vi "Actor Receive.vi"(11 "Dev Actor in":refnum<class "Dev Actor.lvclass">) -> (2 "Msg":refnum<class "Msg Strategy.lvclass">, 3 "Dev Actor out":refnum<class "Dev Actor.lvclass">)   [LabVIEW 2021, in "Dev Actor.lvlib" / "Dev Actor.lvclass"]
uses:
  Dev Actor.lvclass
  <vilib>/jettl/jettl/jettl/Msg Strategy/Msg Strategy.lvclass
  Dev Actor.lvclass/Dev Actor.ctl
  <vilib>/jettl/jettl/jettl/Actor/Actor.lvclass
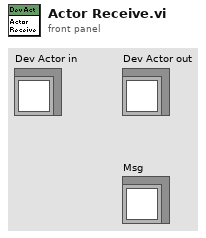
[diagram p1: front panel]
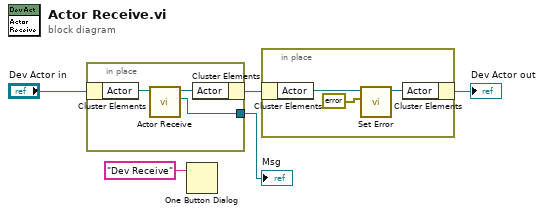
[diagram p0: block diagram]
diagram:
  n1 = in-place {
    in-place-border: [w6] -> w4
    n2 = in-place-cluster #1("Dev Actor in") -> ("Actor"=w8:refnum<class "Actor.lvclass">)
    n3 = call-dynamic "Actor Receive.vi"("Actor in"=w8) -> ("Msg"=w6:refnum<class "Msg Strategy.lvclass">, "Actor out"=w7:refnum<class "Actor.lvclass">)  [unwired: 9 in]
    n4 = in-place-cluster #1("Actor"=w7) -> (w2:refnum<class "Dev Actor.lvclass">)
  }
  "Msg" <- w4
  n5 = One Button Dialog(message="Dev Receive") -> ()  [unwired: 1 in, 1 out]
  n6 = in-place {
    n7 = in-place-cluster #2(w2) -> ("Actor"=w11:refnum<class "Actor.lvclass">)
    n8 = call-dynamic "Set Error.vi"("Error"=errorcluster {"status"=FALSE, "code"=0, "source"=""}, "Actor in"=w11) -> ("Actor out"=w10:refnum<class "Actor.lvclass">)  [unwired: 9 in]
    n9 = in-place-cluster #2("Actor"=w10) -> (→"Dev Actor out":refnum<class "Dev Actor.lvclass">)
  }
